vi "PH_Periodic_Sequencer.set Instances.vi"(0 "i ref in":refnum<vi>, 5 "error in (no error)":errorcluster) -> (14 "i ref out":refnum<vi>, 19 "error out":errorcluster)   [LabVIEW 2014, in "PH_Periodic_Sequencer.lvlib"]
doc: "In this VI all related instances which are not set via the database are named. This is done either hardwired or following naming conventions! Therefore handle with care!"
uses:
  PH_Periodic_Sequencer.lvlib
  PH_Basics/PH_StatusHandler/PH_StatusHandler.Status.ctl
  PH_Basics/PH_StatusHandler/PH_StatusHandler.lvlib
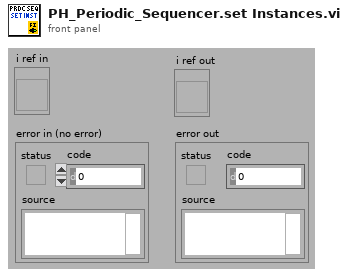
[diagram p1: front panel]
types:
  T1 = typedef "PH_Periodic_Sequencer.lvlib/PH_Periodic_Sequencer.i attribute.ctl" = cluster{"GUI Refs":cluster{"Main Off":refnum<vi>, "Start":refnum<vi>, "Ready":refnum<vi>, "Sequencer SM State":refnum<vi>, "Interval [sec]":refnum<vi>, "Wanted Shots":refnum<vi>, "Delivered Shots":refnum<vi>}, "PU Info":cluster{"Instancename":string, "State":T2, "linked":bool}[], "Sequencer":cluster{"Instancename":string, "linked?":bool, "R2S?":bool, "SM State":string}, "Run?":bool, "Interval [sec]":dbl, "PU State Refs":refnum<vi>[], "Wanted Shots":i32, "Delivered Shots":i32}
  T2 = typedef "PH_StatusHandler.lvlib/PH_StatusHandler.Status.ctl" = i16
  T3 = cluster{"Instancename":string, "State":T2, "linked":bool}
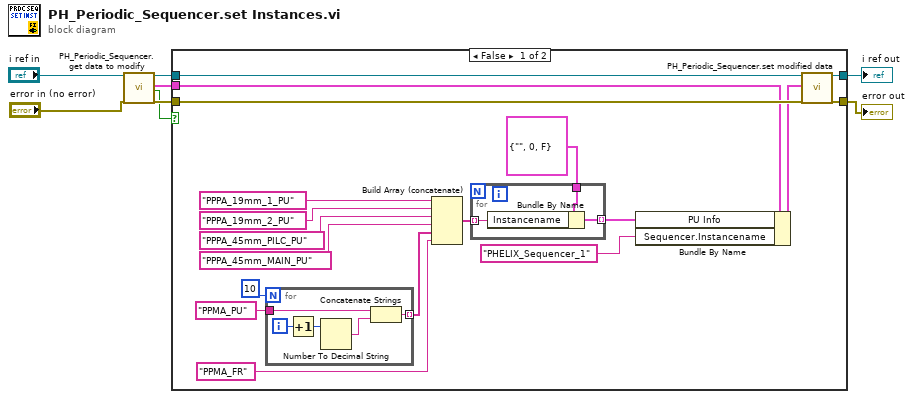
[diagram p0: block diagram]
diagram:
  n1 = call "PH_Periodic_Sequencer.get data to modify.vi"("i ref in"="i ref in", "error in (no error)"="error in (no error)") -> ("i ref out"=w8:refnum<vi>, "i attribute"=w3:T1, "timed out"=w4:bool, "error out"=w6:errorcluster)  [unwired: 14 in]
  n2 = case shown="False" w4 {
    tunnel: w8 -> [w26 w36]
    tunnel: [w25 w36] -> w7
    tunnel: w6 -> [w24 w35]
    tunnel: [w23 w35] -> w5
    tunnel: w3 -> [w21 _]
    frame False {
      n3 = for {
        N: 10 -> [_]
        tunnel: "PPMA_PU" -> [w27]
        tunnel: [w29] -> w19 mode=indexing
        i -> [w31]
        n4 = Increment(x=w31) -> (x+1=w30:i32)
        n5 = Number To Decimal String(number=w30) -> (decimal integer string=w28:string)  [unwired: 1 in]
        n6 = Concatenate Strings(w27, w28) -> (w29:string)
      }
      n7 = Build Array (concatenate) ("PU Instancenames")("PPPA_19mm_1_PU", "PPPA_19mm_2_PU", "PPPA_45mm_PILC_PU", "PPPA_45mm_MAIN_PU", w19, "PPMA_FR") -> (w16:string[])
      n8 = for {
        tunnel: T3 {"Instancename"="", "State"=0, "linked"=FALSE} ("Info PU") -> [w34]
        tunnel: [w33] -> w9 mode=indexing
        tunnel: w16 -> [w32] mode=indexing
        n9 = Bundle By Name(cluster=w34, "Instancename"=w32) -> (w33:T3)
      }
      n10 = Bundle By Name(cluster=w21, "PU Info"=w9, "Sequencer.Instancename"="PHELIX_Sequencer_1") -> (w22:T1)
      n11 = call "PH_Periodic_Sequencer.set modified data.vi"("i ref in"=w26, "i attribute"=w22, "error in (no error)"=w24) -> ("i ref out"=w25:refnum<vi>, "error out"=w23:errorcluster)  [unwired: 15 in]
    }
    frame True {
    }
  }
  "i ref out" <- w7
  "error out" <- w5
